vi "myTask.vi"(8 "error in (no error)":errorcluster, 10 "stopMechanism":refnum<class "ITaskChannel.lvclass">, 11 "ITask in":refnum<class "ITask.lvclass">) -> (0 "error out":errorcluster, 3 "ITask out":refnum<class "ITask.lvclass">)   [LabVIEW 2023, in "Task_BoolUserEventStopMech.lvclass"]
uses:
  Task_BoolUserEventStopMech.lvclass
  ITask/ITask.lvclass
  ITaskChannel/ITaskChannel.lvclass
  C:/projects/TLC_Daemon/source/ITask/ITask.lvclass
  Task_BoolUserEventStopMech.lvclass/Task_BoolUserEventStopMech.ctl
  Read description.vi
  TLC_Daemon.lvlib
  C:/projects/TLC_Daemon/source/Examples/Example_Bool_User_Event_StopMech/Task_BoolUserEventStopMech/Task_BoolUserEventStopMech.lvclass
panel:
  out "loopCounter":i32 caption="Loop Counter"
  out "description":string
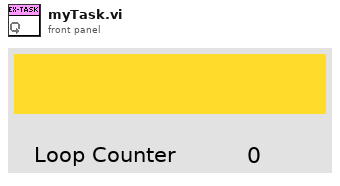
[diagram p1: front panel]
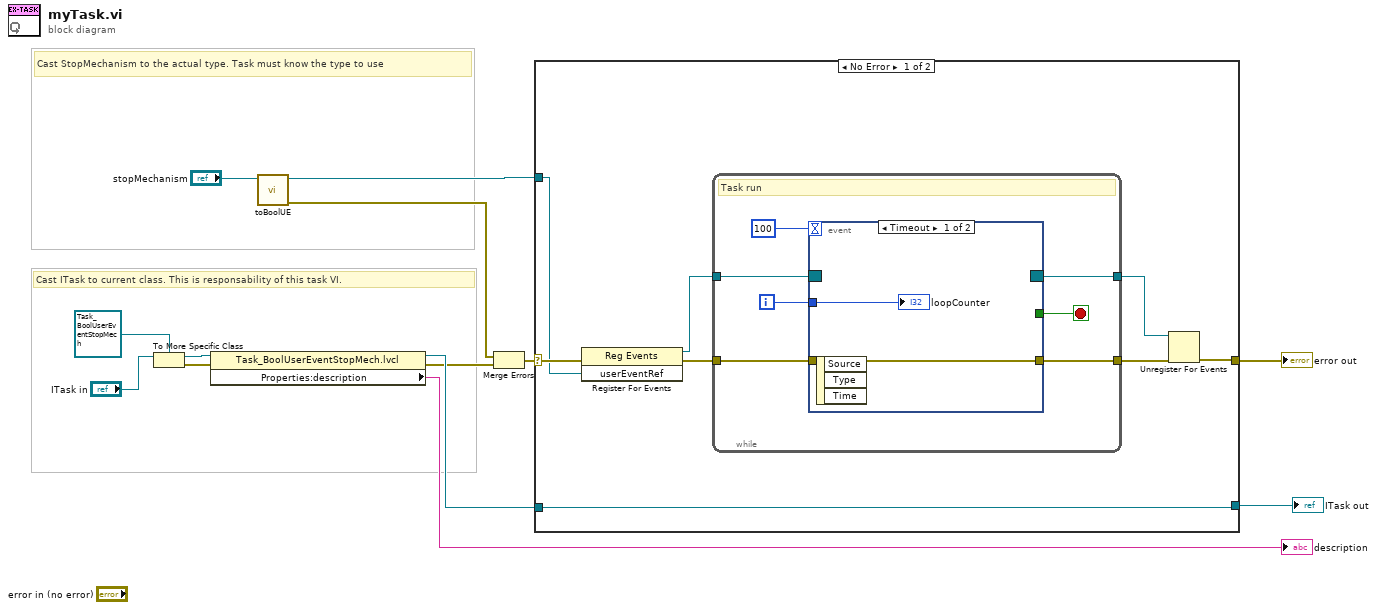
[diagram p0: block diagram]
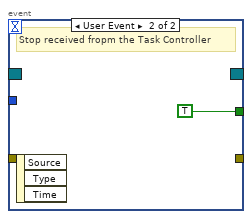
[diagram p2: hidden frame]
diagram:
  # "Cast ITask to current class. This is responsability of this task VI."
  # "Cast StopMechanism to the actual type. Task must know the type to use"
  n1 = To More Specific Class(target class=refnum<class "Task_BoolUserEventStopMech.lvclass"> refnum ("ExampleTask_StopNotifier.lvclass"), reference="ITask in") -> (specific class reference=w10:refnum<class "Task_BoolUserEventStopMech.lvclass">, error out=w11:errorcluster)  [unwired: 1 in]
  n2 = property class="Task_BoolUserEventStopMech.lvcl"(reference=w10, error in=w11) -> (reference out=w8:refnum<class "Task_BoolUserEventStopMech.lvclass">, error out=w6:errorcluster, "Properties:description"=→"description":string)
  n3 = call "toBoolUE.vi"("ITaskChannel"="stopMechanism") -> ("error out"=w1:errorcluster, "userEventRef"=w2:refnum<user-event>)  [unwired: 9 in]
  n4 = Merge Errors(w1, w6) -> (w5:errorcluster)
  n5 = case shown="No Error" w5 {
    selector: w5 -> [w20 w33]
    tunnel: w2 -> [w18 _]
    tunnel: w8 -> [w21 w32]
    tunnel: [w21 w32] -> w7
    tunnel: [w15 w33] -> w4
    frame No Error {
      n6 = register-events(error in=w20, w18) -> (reference out=w17:refnum<event-registration>, error out=w19:errorcluster)  [unwired: 1 in]
      n7 = while {
        tunnel: w19 -> [w28]
        tunnel: [w27] -> w14
        tunnel: w17 -> [w24]
        tunnel: [w22] -> w16
        i -> [w26]
        stop <- w23 stop-if-true
        # "Task run"
        n8 = event shown="[0] Timeout" {
          selector: w24 -> [_ _]
          dyn-events: [_ _] -> w22
          timeout: 100 -> [_ _]
          tunnel: w28 -> [w30 _]
          tunnel: [w30 _] -> w27
          tunnel: w26 -> [w29 _]
          tunnel: [_ TRUE] -> w23
          event Timeout {
            n9 = event-data() -> ()  [unwired: 1 in, 3 out]
            "loopCounter" <- w29
          }
          event User Event {
            # "Stop received fropm the Task Controller"
            n10 = event-data() -> ()  [unwired: 1 in, 3 out]
          }
        }
      }
      n11 = Unregister For Events(event registration refnum=w16, error in=w14) -> (error out=w15:errorcluster)
    }
    frame Error {
    }
  }
  "error out" <- w4
  "ITask out" <- w7
